vi "Grove Digital In.vi"() -> ()   [LabVIEW 2020, in "CTI-Scratchpad.lvlib"]
uses:
  CTI-Scratchpad.lvlib
  CTI/Identity.ctl
  CTI/GPIO Direction.ctl
  CTI/GPIO Number.ctl
  CTI/Session/Session.lvclass
  CTI/CTI.lvlib
  CTI/VisaComms/VisaComms.lvclass
panel:
  out "Boolean 2":bool
  out "Boolean 1":bool
  in  "GroveConnector":enum16{"D16", "D18", "D20"}(ring)
  out "Identity":T1
  in  "Port":refnum<visa-resource-name>="COM6"
  in  "stop":bool
  # "Should Also Work for..."
  # "https://wiki.seeedstudio.com/Grove-Adjustable_PIR_Motion_Sensor/"
  # "https://wiki.seeedstudio.com/Grove-Digital_Distance_Interrupter_0.5_to_5cm-GP2Y0D805Z0F/"
  # "https://wiki.seeedstudio.com/Grove-Flame_Sensor/"
  # "https://wiki.seeedstudio.com/Grove-Hall_Sensor/"
  # "https://wiki.seeedstudio.com/Grove-Infrared_Reflective_Sensor/"
  # "https://wiki.seeedstudio.com/Grove-IR_Distance_Interrupter_v1.2/"
  # "https://wiki.seeedstudio.com/Grove-Line_Finder/"
  # "https://wiki.seeedstudio.com/Grove-Magnetic_Switch/"
  # "https://www.seeedstudio.com/Grove-mini-PIR-motion-sensor-p-2930.html"
  # "https://wiki.seeedstudio.com/Grove-Button/"
  # "https://wiki.seeedstudio.com/Grove-Switch-P/"
  # "https://wiki.seeedstudio.com/Grove-Tilt_Switch/"
  # "https://wiki.seeedstudio.com/Grove-Touch_Sensor/"
  # "https://wiki.seeedstudio.com/Grove-Vibration_Sensor_SW-420/"
  # "https://wiki.seeedstudio.com/Grove-Water_Atomization/"
  # "https://wiki.seeedstudio.com/Grove-Water_Sensor/"
  # "https://www.seeedstudio.com/Grove-Dual-Button-p-4529.html"
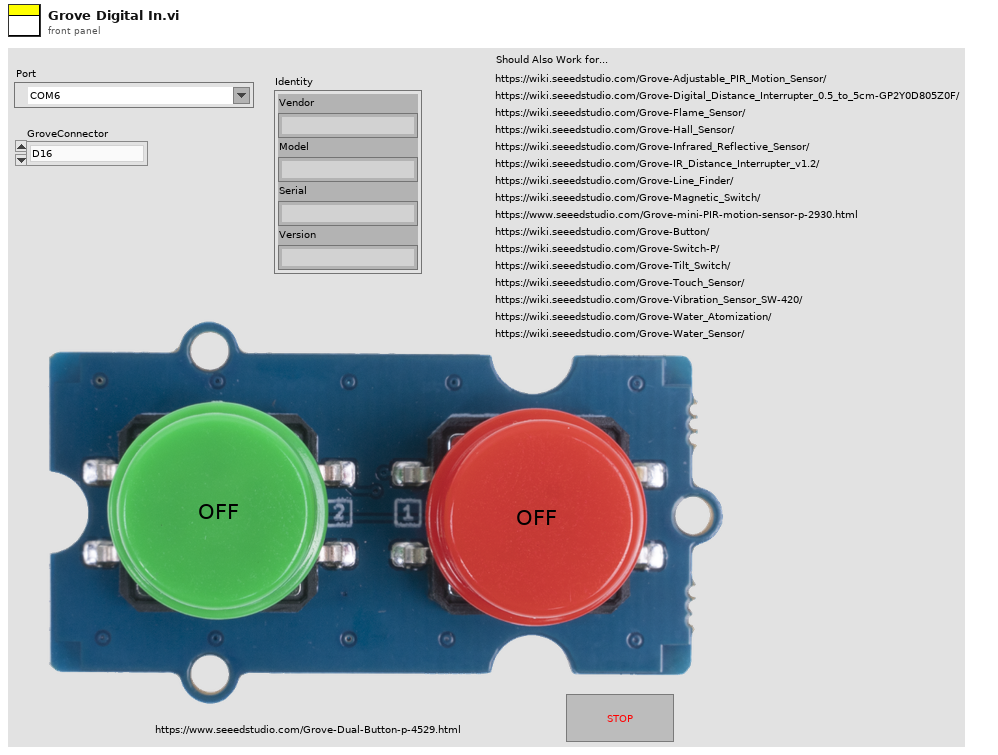
[diagram p1: front panel]
types:
  T1 = typedef "CTI.lvlib/Identity.ctl" = cluster{"Vendor":string, "Model":string, "Serial":string, "Version":string}
  T2 = typedef "CTI.lvlib/GPIO Direction.ctl" = enum16{"In", "Out"}
  T3 = typedef "CTI.lvlib/GPIO Number.ctl" = i8
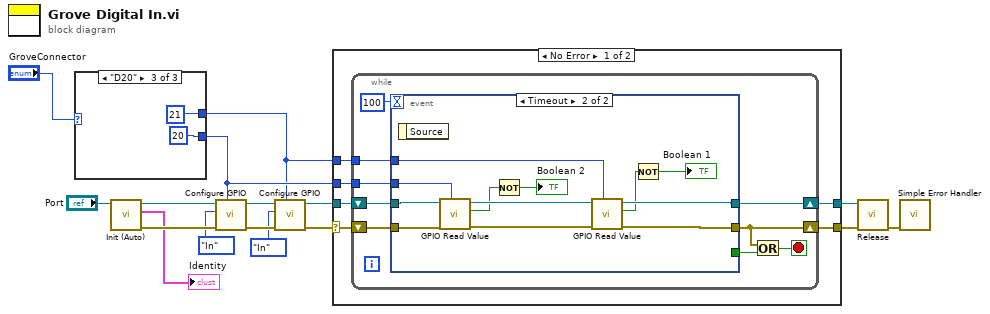
[diagram p0: block diagram]
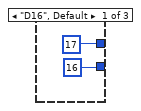
[diagram p2: hidden frame]
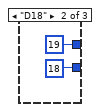
[diagram p3: hidden frame]
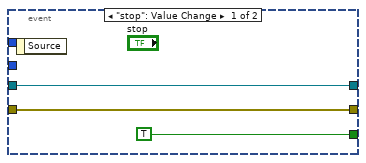
[diagram p4: hidden frame]
diagram:
  n1 = case shown="\"D20\"" "GroveConnector" {
    tunnel: [T3 16 ("GPIO #") T3 18 ("GPIO #") T3 20 ("GPIO #")] -> w7
    tunnel: [T3 17 ("GPIO #") T3 19 ("GPIO #") T3 21 ("GPIO #")] -> w5
    frame "D16", Default {
    }
    frame "D18" {
    }
    frame "D20" {
    }
  }
  n2 = call "Init (Auto).vi"("VISA resource name"="Port") -> ("error out"=w14:errorcluster, "Identity"=→"Identity":T1, "Session"=w15:refnum<class "Session.lvclass">)  [unwired: 8 in]
  n3 = call "Configure GPIO.vi"("GPIO #"=w7, "error in (no error)"=w14, "GPIO Direction"=GPIO_Direction."In", "Session in"=w15) -> ("error out"=w6:errorcluster, "Session out"=w4:refnum<class "Session.lvclass">)  [unwired: 6 in]
  n4 = call "Configure GPIO.vi"("GPIO #"=w5, "error in (no error)"=w6, "GPIO Direction"=GPIO_Direction."In", "Session in"=w4) -> ("error out"=w2:errorcluster, "Session out"=w3:refnum<class "Session.lvclass">)  [unwired: 6 in]
  n5 = case shown="No Error" w2 {
    selector: w2 -> [w27 w53]
    tunnel: w3 -> [w28 w54]
    tunnel: [w26 w54] -> w11
    tunnel: [w25 w53] -> w13
    tunnel: w7 -> [w24 _]
    tunnel: w5 -> [w23 _]
    frame No Error {
      n6 = while {
        shift-right: [w35] -> w26
        shift-left: w28 -> [w37]
        shift-right: [w34] -> w25
        shift-left: w27 -> [w36]
        tunnel: w24 -> [w31]
        tunnel: w23 -> [w30]
        stop <- w33 stop-if-true
        n7 = event shown="[1] Timeout" {
          selector: _ -> [_ _]
          dyn-events: _ -> [_ _]
          timeout: 100 -> [_ _]
          tunnel: w37 -> [w40 w50]
          tunnel: w36 -> [w39 w49]
          tunnel: [w40 w46] -> w35
          tunnel: [w39 w45] -> w34
          tunnel: [TRUE _] -> w32
          tunnel: w31 -> [_ w48]
          tunnel: w30 -> [_ w47]
          event "stop": Value Change {
            n8 = event-data() -> ()  [unwired: 1 in, 1 out]
          }
          event Timeout {
            n9 = event-data() -> ()  [unwired: 1 in, 1 out]
            n10 = call "GPIO Read Value.vi"("GPIO #"=w48, "error in (no error)"=w49, "Session in"=w50) -> ("error out"=w51:errorcluster, "Value"=w43:bool, "Session out"=w52:refnum<class "Session.lvclass">)  [unwired: 6 in]
            n11 = Not(x=w43) -> (.not. x?=→"Boolean 2":bool)
            n12 = call "GPIO Read Value.vi"("GPIO #"=w47, "error in (no error)"=w51, "Session in"=w52) -> ("error out"=w45:errorcluster, "Value"=w44:bool, "Session out"=w46:refnum<class "Session.lvclass">)  [unwired: 6 in]
            n13 = Not(x=w44) -> (.not. x?=→"Boolean 1":bool)
          }
        }
        n14 = Or(x=w34, y=w32) -> (x .or. y?=w33:bool)
      }
    }
    frame Error {
    }
  }
  n15 = call-dynamic "Release.vi"("error in (no error)"=w13, "Session in"=w11) -> ("error out"=w12:errorcluster)  [unwired: 9 in]
  n16 = call <vilib>:"Simple Error Handler.vi"("error in (no error)"=w12) -> ()  [unwired: 4 in, 5 out]
